vi "TTL_test.vi"() -> ()   [LabVIEW 2013, in "TTL_input.lvclass"]
uses:
  TTL_input.lvclass
  <vilib>/Utility/error.llb/DialogType.ctl
  <vilib>/DAQmx/read.llb/DAQmx Read (Digital 1D Bool 1Chan 1Samp).vi
  <vilib>/DAQmx/create/channels.llb/DAQmx Create Channel (DI-Digital Input).vi
  <vilib>/DAQmx/miscellaneous.llb/DAQmx Fill In Error Info.vi
  <vilib>/DAQmx/configure/timing.llb/DAQmx Timing (Sample Clock).vi
panel:
  out "data":bool[](array[boolean])
  in  "lines":tag="PXI1Slot6/port1/line1:2"
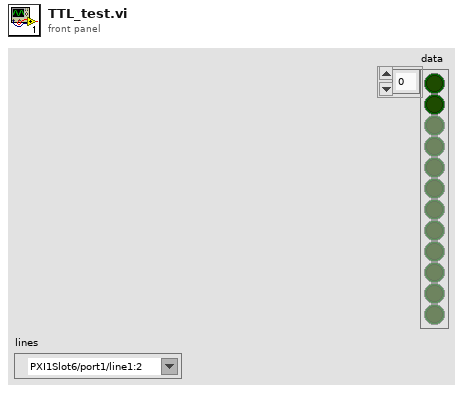
[diagram p1: front panel]
types:
  T1 = typedef "DialogType.ctl" = u16
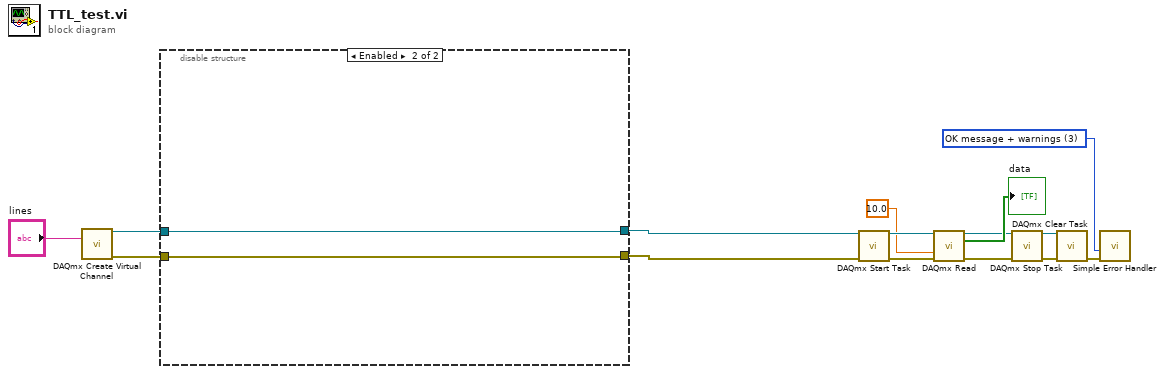
[diagram p0: block diagram]
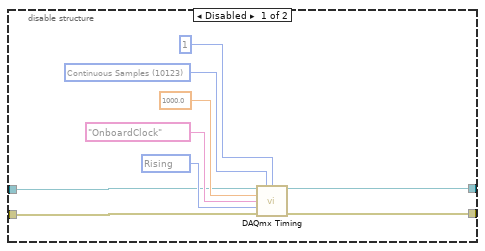
[diagram p2: hidden frame]
diagram:
  w5 = T1 3 items=["no dialog", "OK message", "continue or stop message", "OK message + warnings", "continue/stop + warnings"] ("type of dialog (OK msg:1)")
  n1 = call-poly <vilib>:"DAQmx Create Virtual Channel.vi"("lines"="lines") -> ("task out"=w2:refnum<k21>, "error out"=w4:errorcluster)  [unwired: 13 in]
  n2 = disable-structure shown="Enabled" {
    disable-tunnel: w4 -> [w19 w25]
    disable-tunnel: [w18 w25] -> w3
    disable-tunnel: w2 -> [w17 w26]
    disable-tunnel: [w16 w26] -> w1
    frame Disabled {
      w20 = 10280 items=["Rising"=10280, "Falling"=10171] ("active edge")
      w23 = 10123 items=["Finite Samples"=10178, "Continuous Samples"=10123, "Hardware Timed Single Point"=12522] ("sample mode")
      n3 = call-poly <vilib>:"DAQmx Timing.vi"("task/channels in"=w17, "sample mode"=w23, "samples per channel"=1, "rate"=1000.0, "source"=tag "OnboardClock", "active edge"=w20, "error in"=w19) -> ("task out"=w16:refnum<k21>, "error out"=w18:errorcluster)  [unwired: 7 in]
    }
    frame Enabled {
    }
  }
  n4 = call <vilib>:"DAQmx Start Task.vi"("task/channels in"=w1, "error in"=w3) -> ("task out"=w13:refnum<k21>, "error out"=w14:errorcluster)  [unwired: 12 in]
  n5 = call-poly <vilib>:"DAQmx Read.vi"("task/channels in"=w13, "timeout"=10.0, "error in"=w14) -> ("task out"=w10:refnum<k21>, "data"=→"data":bool[], "error out"=w11:errorcluster)  [unwired: 10 in]
  n6 = call <vilib>:"DAQmx Stop Task.vi"("task/channels in"=w10, "error in"=w11) -> ("task out"=w7:refnum<k21>, "error out"=w8:errorcluster)  [unwired: 12 in]
  n7 = call <vilib>:"DAQmx Clear Task.vi"("task in"=w7, "error in"=w8) -> ("error out"=w6:errorcluster)  [unwired: 13 in]
  n8 = call <vilib>:"Simple Error Handler.vi"("type of dialog (OK msg:1)"=w5, "error in (no error)"=w6) -> ()  [unwired: 3 in, 5 out]
